vi "SetActiveGraphic.vi"(4 "Shift":bool, 6 "CTRL?":bool, 8 "error in (no error)":errorcluster, 9 "Active Layer":i32, 10 "Ctl Refnum":refnum<vi>, 11 "FakedArray in":refnum<class "FakedArray.lvclass">) -> (0 "error out":errorcluster, 3 "FakedArray out":refnum<class "FakedArray.lvclass">)   [LabVIEW 2021, in "FakedArray.lvclass"]
uses:
  <resource>/plugins/NIIconEditor/Class/FakedArray/FakedArray.lvclass
  <resource>/plugins/NIIconEditor/Class/FakedArray/FakedArray.lvclass/FakedArray.ctl
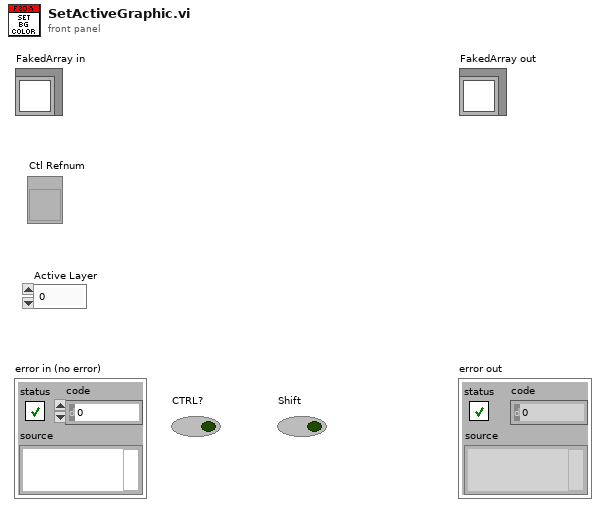
[diagram p1: front panel]
types:
  T1 = typedef "IEColor.ctl" = u32
  T2 = typedef "ToMoreSpecific_Faked2DArray.ctl" = enum16{"Framework Templates", "Layer List"}
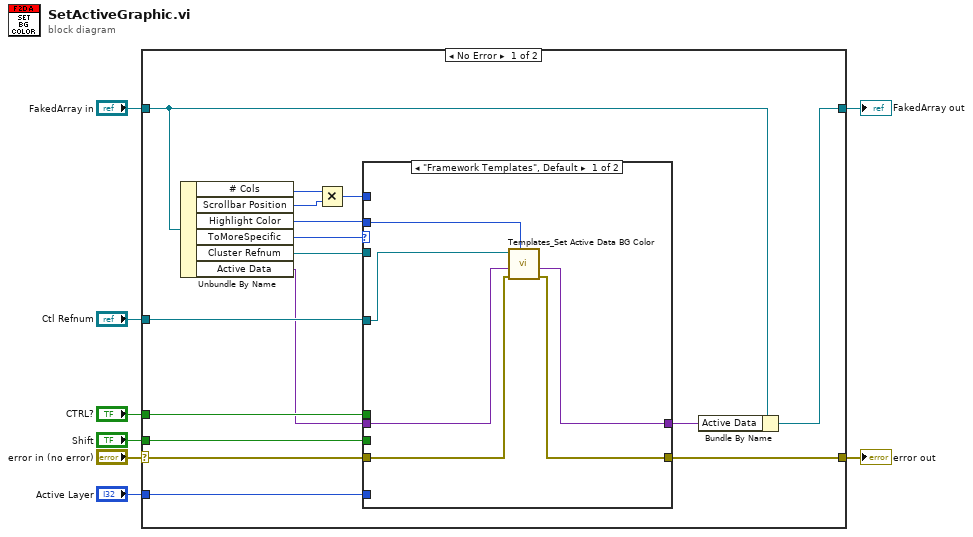
[diagram p0: block diagram]
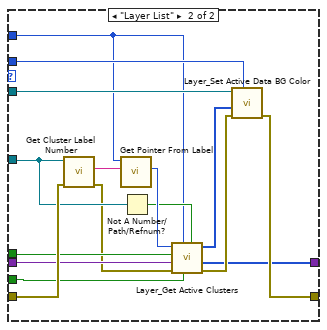
[diagram p2: hidden frame]
diagram:
  n1 = case shown="No Error" "error in (no error)" {
    selector: "error in (no error)" -> [w24 w48]
    tunnel: [w23 w48] -> w7
    tunnel: [w19 w47] -> w5
    tunnel: "FakedArray in" -> [w22 w47]
    tunnel: "Ctl Refnum" -> [w17 _]
    tunnel: "Active Layer" -> [w15 _]
    tunnel: "CTRL?" -> [w13 _]
    tunnel: "Shift" -> [w9 _]
    frame No Error {
      n2 = Unbundle By Name(w22) -> ("# Cols"=w10:i32, "Scrollbar Position"=w14:i32, "Highlight Color"=w20:T1, "ToMoreSpecific"=w21:T2, "Cluster Refnum"=w16:refnum<vi>, "Active Data"=w12:variant)
      n3 = Multiply(x=w10, y=w14) -> (x*y=w11:i32)
      n4 = case shown="\"Framework Templates\", Default" w21 {
        tunnel: w17 -> [w25 w41]
        tunnel: w24 -> [w29 w46]
        tunnel: [w26 w34] -> w23
        tunnel: w20 -> [w30 w37]
        tunnel: [w27 w33] -> w18
        tunnel: w16 -> [_ w38]
        tunnel: w15 -> [_ _]
        tunnel: w13 -> [_ w43]
        tunnel: w12 -> [w28 w44]
        tunnel: w11 -> [_ w32]
        tunnel: w9 -> [_ w31]
        frame "Framework Templates", Default {
          n5 = call <resource>:"Templates_Set Active Data BG Color.vi"("Highlight Color"=w30, "error in"=w29, "Active Data"=w28, "Ctl Refnum"=w25) -> ("error out"=w26:errorcluster, "Active Data"=w27:variant)  [unwired: 6 out]
        }
        frame "Layer List" {
          n6 = call <resource>:"Get Cluster Label Number.vi"("error in"=w46, "Ref in"=w41) -> ("error out"=w36:errorcluster, "Label.Text"=w45:string)  [unwired: 8 out]
          n7 = call <resource>:"Get Pointer From Label.vi"("Label"=w45, "Offset"=w32) -> ("Absolut Pointer"=w42:u32)  [unwired: 9 out]
          n8 = Not A Number/Path/Refnum?(number/path/refnum=w41) -> (NaN/Path/Refnum?=w40:bool)
          n9 = call <resource>:"Layer_Get Active Clusters.vi"("Get active Data only?"=w40, "Shift?"=w31, "Offset"=w32, "error in"=w36, "Active Data"=w44, "CTRL?"=w43, "Absolut Pointer"=w42) -> ("error out"=w35:errorcluster, "Active Data out"=w33:u32[], "Relative Indices []"=w39:u32[])  [unwired: 2 out]
          n10 = call <resource>:"Layer_Set Active Data BG Color.vi"("Highlight Color"=w37, "error in"=w35, "Highlighted Indices"=w39, "Cluster Refnum"=w38) -> ("error out"=w34:errorcluster)  [unwired: 7 out]
        }
      }
      n11 = Bundle By Name(cluster=w22, "Active Data"=w18) -> (w19:refnum<class "FakedArray.lvclass">)
    }
    frame Error {
    }
  }
  "error out" <- w7
  "FakedArray out" <- w5
